vi "RequestStreaming RouteGuide Test.vi"() -> ()   [LabVIEW 2019, in "route_guide_client.lvlib"]
uses:
  route_guide_client.lvlib
  RPC Messages/routeguide_RouteSummary.ctl
  <vilib>/gRPC/LabVIEW gRPC Library/grpc-lvsupport-release.lvlib
panel:
  out "error out":errorcluster
  in  "ms per iteration":u32=200
  in  "Longitude Loop":i32=4
  in  "Latitude Loop":i32=4
  out "Response Data":T1
  in  "Server Address":string="localhost:50051"
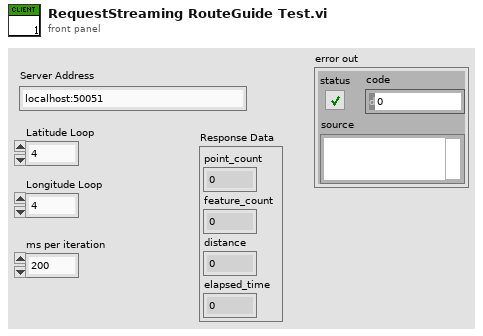
[diagram p1: front panel]
types:
  T1 = typedef "route_guide_client.lvlib/routeguide_RouteSummary.ctl" = cluster{"point_count":i32, "feature_count":i32, "distance":i32, "elapsed_time":i32}
  T2 = typedef "grpc-lvsupport-release.lvlib/grpcId.ctl" = u64
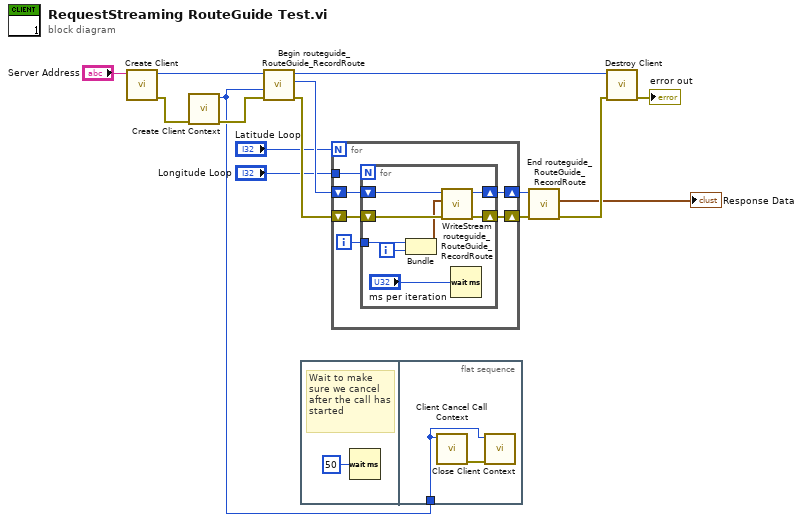
[diagram p0: block diagram]
diagram:
  n1 = call "Create Client.vi"("address"="Server Address") -> ("error out"=w4:errorcluster, "gRPC ID Out"=w14:T2)  [unwired: 9 in]
  n2 = call <vilib>:"Create Client Context.vi"("error in (no error)"=w4) -> ("error out"=w3:errorcluster, "ContextID out"=w2:T2)  [unwired: 9 in]
  n3 = call "Begin routeguide_RouteGuide_RecordRoute.vi"("error in"=w3, "contextId"=w2, "gRPC ID"=w14) -> ("error out"=w12:errorcluster, "Call Id Out"=w13:T2, "gRPC ID out"=w8:T2)  [unwired: 6 in]
  n4 = flat-sequence {
    tunnel: w2 -> [w17]
    frame #0 {
      # "Wait to make sure we cancel after the call has started"
      n5 = Wait (ms)(milliseconds to wait=u32 50) -> ()  [unwired: 1 out]
    }
    frame #1 {
      n6 = call <vilib>:"Client Cancel Call Context.vi"("Call ID in"=w17) -> ("error out"=w18:errorcluster)  [unwired: 10 in]
      n7 = call <vilib>:"Close Client Context.vi"("error in (no error)"=w18, "ContextID"=w17) -> ()  [unwired: 9 in, 1 out]
    }
  }
  n8 = for {
    N: "Latitude Loop" -> [_]
    shift-right: [w21] -> w10
    shift-left: w13 -> [w24]
    shift-right: [w22] -> w11
    shift-left: w12 -> [w23]
    tunnel: "Longitude Loop" -> [w19]
    i -> [w20]
    n9 = for {
      N: w19 -> [_]
      shift-right: [w29] -> w21
      shift-left: w24 -> [w32]
      shift-right: [w30] -> w22
      shift-left: w23 -> [w31]
      tunnel: w20 -> [w26]
      i -> [w28]
      n10 = Bundle(w26, w28) -> (w27:cluster{i32, i32})  [unwired: 1 in]
      n11 = call "WriteStream routeguide_RouteGuide_RecordRoute.vi"("error in"=w31, "Request Data"=w27, "Call ID in"=w32) -> ("error out"=w30:errorcluster, "Call ID"=w29:T2)  [unwired: 6 in, 1 out]
      n12 = Wait (ms)(milliseconds to wait="ms per iteration") -> ()  [unwired: 1 out]
    }
  }
  n13 = call "End routeguide_RouteGuide_RecordRoute.vi"("error in"=w11, "Call ID in"=w10) -> ("error out"=w9:errorcluster, "Response Data"=→"Response Data":T1)  [unwired: 7 in, 1 out]
  n14 = call "Destroy Client.vi"("error in"=w9, "gRPC ID"=w8) -> ("error out"=→"error out":errorcluster)  [unwired: 9 in]
